vi "Write Sinusoid Stimulus Parameter.vi"(8 "error in (no error)":errorcluster, 10 "Stimulus Parameters":T1, 11 "Data Analyser Report in":refnum<class "Data Analyser Report.lvclass">) -> (0 "error out":errorcluster, 3 "Data Analyser Report out":refnum<class "Data Analyser Report.lvclass">)   [LabVIEW 2016, in "Data Analyser Report.lvclass"]
uses:
  Data Analyser Report.lvclass
  C:/Users/w.figtree/Desktop/Work/4. Projects/3. In Progress Engineering Projects/EMA/src/core/Classes/Excel Interface/Excel Sheet/Excel Sheet.lvclass
  Excel Interface/Excel Sheet/Write to Cell - Dbl.vi
  Excel Interface/Excel Sheet/Write to Cell - Int.vi
  Excel Interface/Excel Sheet/Excel Sheet.lvclass
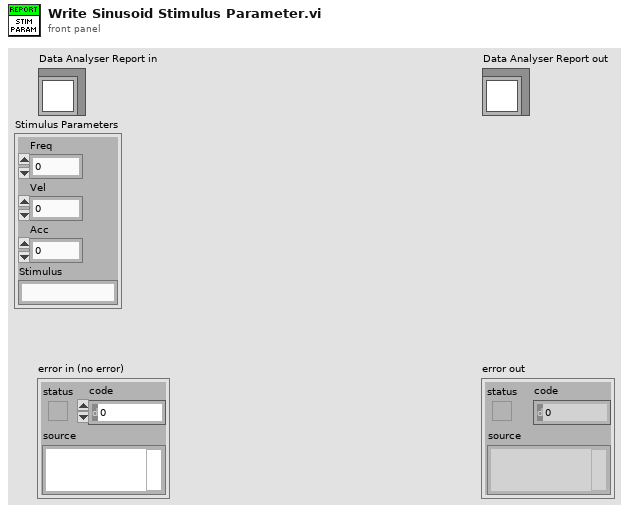
[diagram p1: front panel]
types:
  T1 = cluster{"Freq":dbl, "Vel":i32, "Acc":i32, "Stimulus":string}
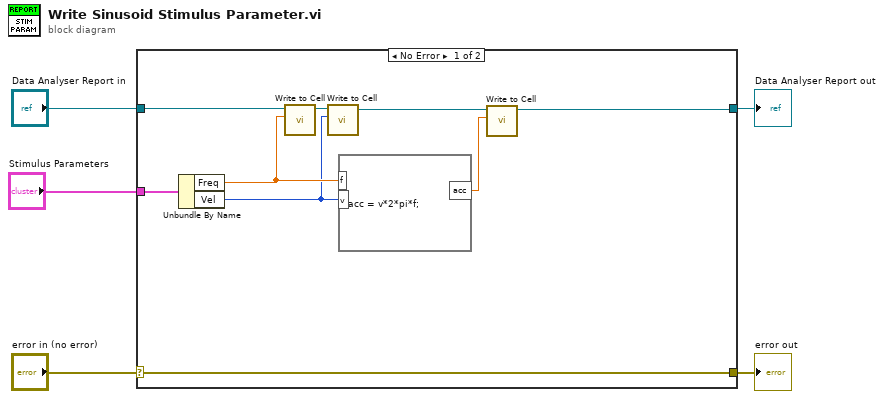
[diagram p0: block diagram]
diagram:
  n1 = case shown="No Error" "error in (no error)" {
    selector: "error in (no error)" -> [w14 w16]
    tunnel: [w14 w16] -> w4
    tunnel: [w9 w15] -> w2
    tunnel: "Data Analyser Report in" -> [w12 w15]
    tunnel: "Stimulus Parameters" -> [w13 _]
    frame No Error {
      n2 = Unbundle By Name(w13) -> ("Freq"=w11:dbl, "Vel"=w10:i32)
      n3 = call-poly "Write to Cell.vi"("Value"=w11, "Excel Sheet in"=w12) -> ("Excel Sheet out"=w8:refnum<class "Data Analyser Report.lvclass">)  [unwired: 9 in]
      n4 = call-poly "Write to Cell.vi"("Value"=w10, "Excel Sheet in"=w8) -> ("Excel Sheet out"=w6:refnum<class "Data Analyser Report.lvclass">)  [unwired: 9 in]
      n5 = formula code="acc = v*2*pi*f;"("v"=w10, "f"=w11) -> ("acc"=w7:dbl)
      n6 = call-poly "Write to Cell.vi"("Value"=w7, "Excel Sheet in"=w6) -> ("Excel Sheet out"=w9:refnum<class "Data Analyser Report.lvclass">)  [unwired: 9 in]
    }
    frame Error {
    }
  }
  "error out" <- w4
  "Data Analyser Report out" <- w2
